vi "main.vi"() -> ()   [LabVIEW 2021]
uses:
  <vilib>/httpClient/LabVIEWHTTPClient.lvlib
  <vilib>/Analysis/NI_AALBase.lvlib
panel:
  out "数组":dbl[](array[numeric])
  in  "管理界面":bool
  in  "退出系统":bool
  in  "登录界面":bool
  in  "主界面":bool
  in  "选项卡":enum32{"主界面", "管理界面", "登录界面"}(tab)
  out "液位高度":dbl format="%#.1f"
  in  "请输入测量点高度":dbl
  out "测量点至水面距离":dbl format="%#.1f"
  in  "开关":bool
  out "液位过低":bool
  out "液位曲线图":dbl(graph)
  out "液位过高":bool
  out "实时液位":dbl(slide) scale=0.0..1000.0
  in  "密码组":string[](array[string])=["001", "002", "003"]
  in  "取消按钮":bool
  in  "登录按钮":bool=TRUE
  in  "密码":string
  in  "用户":enum16{"操作员", "管理员", "开发者"}(ring)
  # "超声波液位测量系统\n超声波液位测量系统"
  # "mm"
  # "mm"
  # "mm"
  # "mm"
  # "操作员"
  # "管理员"
  # "开发者"
  # "用户"
  # "密码"
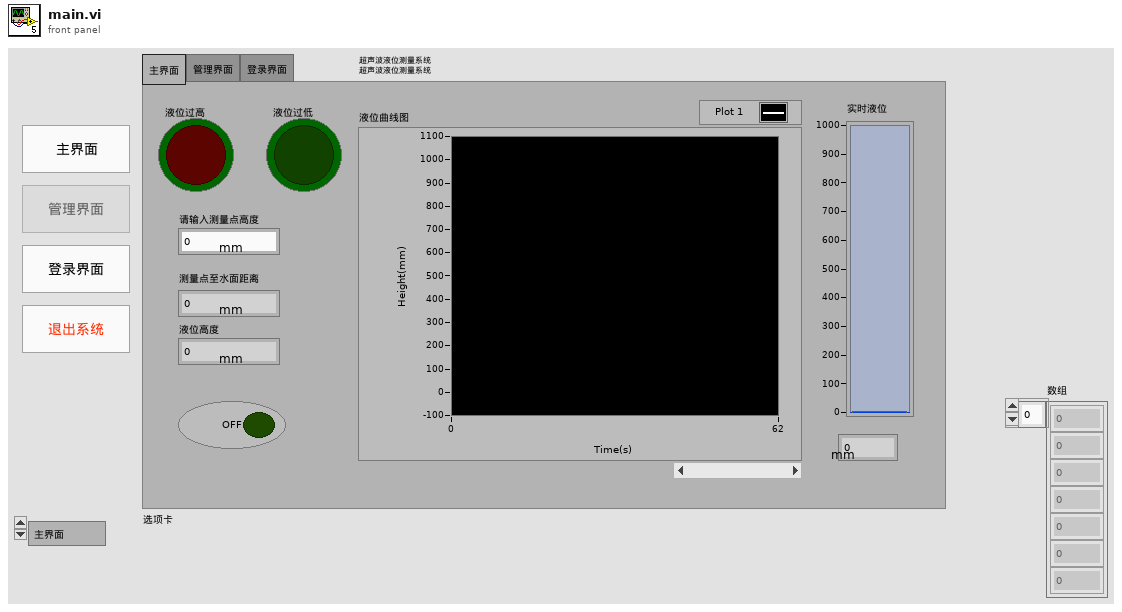
[diagram p1: front panel]
types:
  T1 = enum8{"Enabled", "Disabled", "Disabled and Grayed Out"}
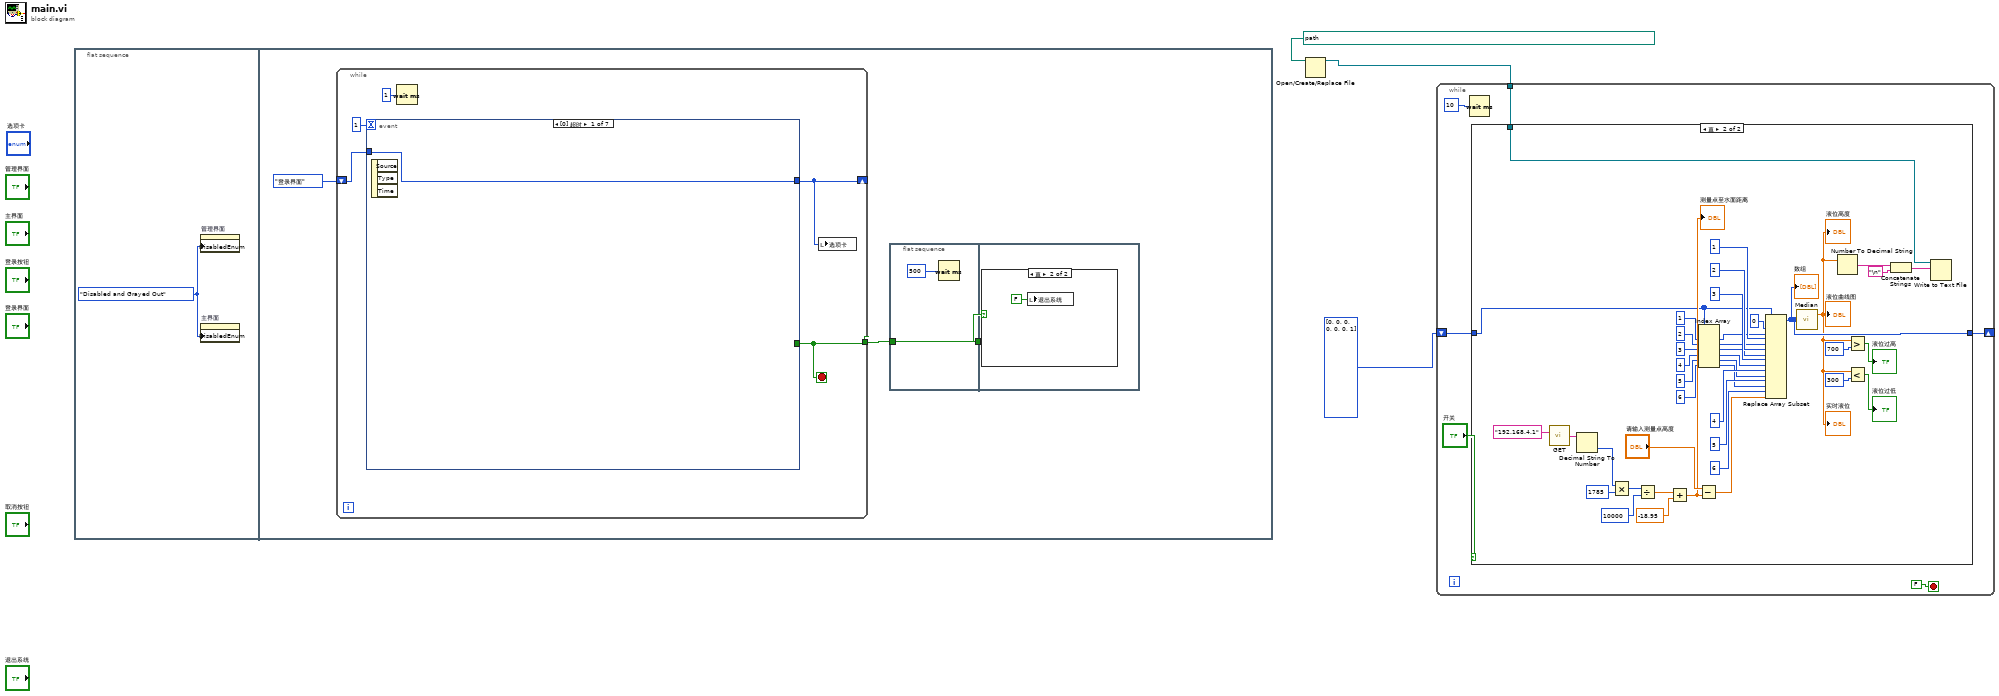
[diagram p0: block diagram]
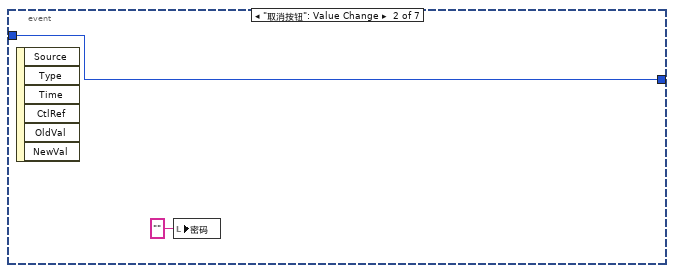
[diagram p4: hidden frame]
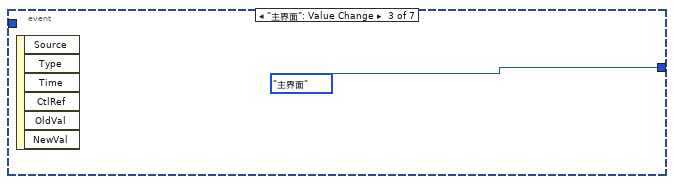
[diagram p5: hidden frame]
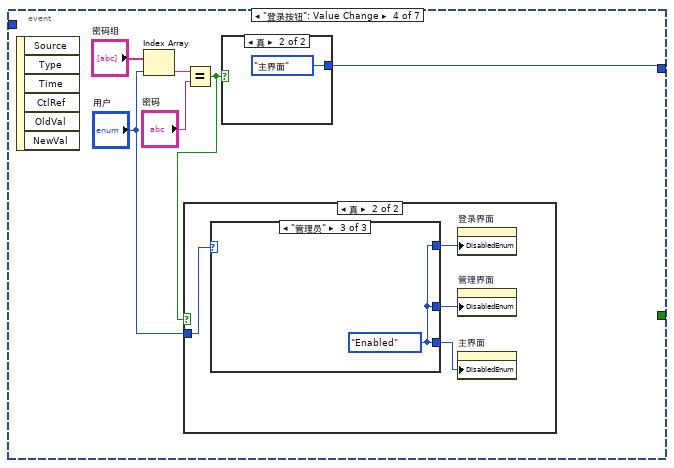
[diagram p6: hidden frame]
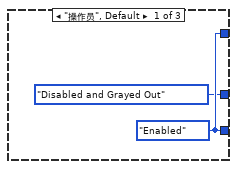
[diagram p8: hidden frame]
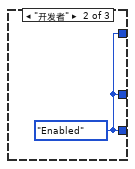
[diagram p9: hidden frame]
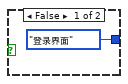
[diagram p10: hidden frame]
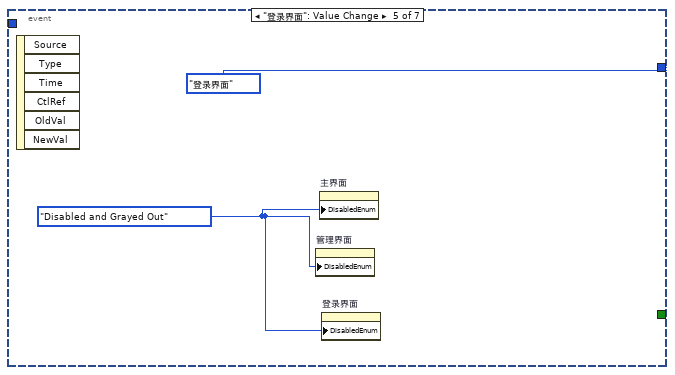
[diagram p11: hidden frame]
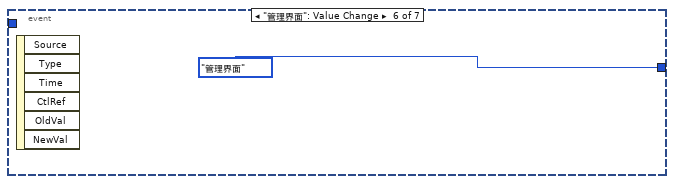
[diagram p12: hidden frame]
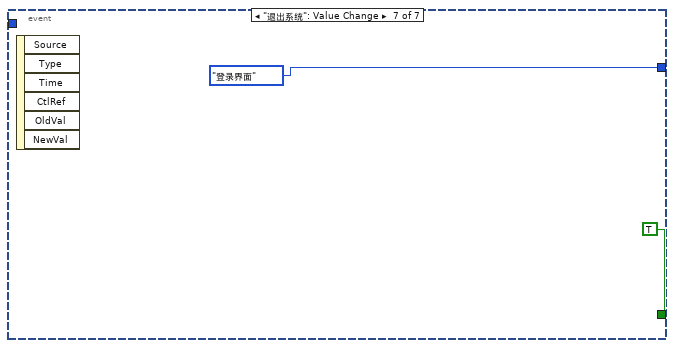
[diagram p13: hidden frame]
diagram:
  n1 = flat-sequence {
    frame #0 {
      w4 = T1."Disabled and Grayed Out" ("禁用")
      n2 = property on="管理界面" class="Bool (严格)"("DisabledEnum"=w4) -> ()  [unwired: 2 in, 2 out]
      n3 = property on="主界面" class="Bool (严格)"("DisabledEnum"=w4) -> ()  [unwired: 2 in, 2 out]
    }
    frame #1 {
      n4 = while {
        shift-right: [w12] -> _
        shift-left: enum32{"主界面", "管理界面", "登录界面"}."登录界面" ("选项卡") -> [w14]
        tunnel: [w13] -> w6
        stop <- w13 stop-if-true
        n5 = event shown="[0] 超时" {
          selector: _ -> [_ _ _ _ _ _ _]
          dyn-events: _ -> [_ _ _ _ _ _ _]
          timeout: 1 -> [_ _ _ _ _ _ _]
          tunnel: w14 -> [w17 w18 _ _ _ _ _]
          tunnel: [w17 w18 enum32{"主界面", "管理界面", "登录界面"}."主界面" ("选项卡") w23 enum32{"主界面", "管理界面", "登录界面"}."登录界面" ("选项卡") enum32{"主界面", "管理界面", "登录界面"}."管理界面" ("选项卡") enum32{"主界面", "管理界面", "登录界面"}."登录界面" ("选项卡")] -> w12
          tunnel: [_ _ _ _ _ _ TRUE] -> w13
          event Timeout {
            n6 = event-data() -> ()  [unwired: 1 in, 3 out]
          }
          event "取消按钮": Value Change {
            n7 = event-data() -> ()  [unwired: 1 in, 6 out]
            n8 = local write "密码"("" ("密码")) -> ()
          }
          event "主界面": Value Change {
            n9 = event-data() -> ()  [unwired: 1 in, 6 out]
          }
          event "登录按钮": Value Change {
            n10 = event-data() -> ()  [unwired: 1 in, 6 out]
            n11 = Index Array(array="密码组", index="用户") -> (element=w25:string)
            n12 = Equal?(x=w25, y="密码") -> (x = y?=w21:bool)
            n13 = case shown="真" w21 {
              tunnel: "用户" -> [_ w30]
              frame False {
              }
              frame True {
                n14 = case shown="\"管理员\"" w30 {
                  tunnel: [w32 w33 w34] -> w29
                  tunnel: [w32 w33 w34] -> w28
                  tunnel: [T1."Disabled and Grayed Out" ("禁用") w33 w34] -> w27
                  frame "操作员", Default {
                    w32 = T1."Enabled" ("禁用")
                  }
                  frame "开发者" {
                    w33 = T1."Enabled" ("禁用")
                  }
                  frame "管理员" {
                    w34 = T1."Enabled" ("禁用")
                  }
                }
                n15 = property on="登录界面" class="Bool (严格)"("DisabledEnum"=w28) -> ()  [unwired: 2 in, 2 out]
                n16 = property on="管理界面" class="Bool (严格)"("DisabledEnum"=w27) -> ()  [unwired: 2 in, 2 out]
                n17 = property on="主界面" class="Bool (严格)"("DisabledEnum"=w29) -> ()  [unwired: 2 in, 2 out]
              }
            }
            n18 = case shown="真" w21 {
              tunnel: [enum32{"主界面", "管理界面", "登录界面"}."登录界面" ("选项卡") enum32{"主界面", "管理界面", "登录界面"}."主界面" ("选项卡")] -> w23
              frame False {
              }
              frame True {
              }
            }
          }
          event "登录界面": Value Change {
            w37 = T1."Disabled and Grayed Out" ("禁用")
            n19 = event-data() -> ()  [unwired: 1 in, 6 out]
            n20 = property on="管理界面" class="Bool (严格)"("DisabledEnum"=w37) -> ()  [unwired: 2 in, 2 out]
            n21 = property on="主界面" class="Bool (严格)"("DisabledEnum"=w37) -> ()  [unwired: 2 in, 2 out]
            n22 = property on="登录界面" class="Bool (严格)"("DisabledEnum"=w37) -> ()  [unwired: 2 in, 2 out]
          }
          event "管理界面": Value Change {
            n23 = event-data() -> ()  [unwired: 1 in, 6 out]
          }
          event "退出系统": Value Change {
            n24 = event-data() -> ()  [unwired: 1 in, 6 out]
          }
        }
        n25 = Wait (ms)(milliseconds to wait=u32 1 ("等待时间（毫秒）")) -> ()  [unwired: 1 out]
        n26 = local write "选项卡"(w12) -> ()
      }
      n27 = flat-sequence {
        tunnel: w6 -> [w9]
        tunnel: [w9] -> w7
        tunnel: w7 -> [w10]
        frame #0 {
          n28 = Wait (ms)(milliseconds to wait=u32 500 ("毫秒计时值")) -> ()  [unwired: 1 out]
        }
        frame #1 {
          n29 = case shown="真" w10 {
            frame False {
            }
            frame True {
              n30 = local write "退出系统"(FALSE ("退出系统")) -> ()
            }
          }
        }
      }
    }
  }
  n31 = Open/Create/Replace File(file path (use dialog)=path "D:/Users/.comberdare/Desktop/超声波测量系统 文件夹/超声波测量系统 文件夹/Database.txt") -> (refnum out=w2:refnum<file>)  [unwired: 5 in, 2 out]
  n32 = while {
    tunnel: w2 -> [w44]
    shift-right: [w42] -> _
    shift-left: i32[] [0, 0, 0, 0, 0, 0, 1] -> [w43]
    stop <- FALSE stop-if-true
    n33 = Wait (ms)(milliseconds to wait=u32 10) -> ()  [unwired: 1 out]
    n34 = case shown="真" "开关" {
      tunnel: w44 -> [_ w89]
      tunnel: w43 -> [w48 w61]
      tunnel: [w48 w53] -> w42
      frame False {
      }
      frame True {
        n35 = call <vilib>:"GET.vi"("url"="192.168.4.1") -> ("body"=w51:string)  [unwired: 11 in, 3 out]
        n36 = Decimal String To Number(string=w51) -> (number=w49:i32)  [unwired: 2 in, 1 out]
        n37 = Multiply(x=w49, y=1785) -> (x*y=w86:i32)
        n38 = Divide(x=w86, y=10000) -> (x/y=w84:dbl)
        n39 = Add(x=w84, y=-18.95) -> (x+y=w82:dbl)
        "测量点至水面距离" <- w82
        n40 = Subtract(x="请输入测量点高度", y=w82) -> (x-y=w62:dbl)
        n41 = Index Array(array=w61, index #1=1 ("索引"), index #2=2 ("索引"), index #3=3 ("索引"), index #4=4 ("索引"), index #5=5 ("索引"), index #6=6 ("索引")) -> (element #1=w68:i32, element #2=w67:i32, element #3=w66:i32, element #4=w65:i32, element #5=w64:i32, element #6=w63:i32)
        n42 = Replace Array Subset(array=w61, new element #1=w68, index #1=0 ("索引"), new element #2=w67, index #2=1 ("索引"), new element #3=w66, index #3=2 ("索引"), new element #4=w65, index #4=3 ("索引"), new element #5=w64, index #5=4 ("索引"), new element #6=w63, index #6=5 ("索引"), new element #7=w62, index #7=6 ("索引")) -> (w53:i32[])
        "数组" <- w53
        n43 = call <vilib>:"Median.vi"("X"=w53) -> ("median"=w52:dbl)  [unwired: 1 out]
        "液位曲线图" <- w52
        "实时液位" <- w52
        "液位高度" <- w52
        n44 = Number To Decimal String(number=w52) -> (decimal integer string=w54:string)  [unwired: 1 in]
        n45 = Greater?(x=w52, y=700) -> (0:→"液位过高":bool)
        n46 = Less?(x=w52, y=300) -> (x < y?=→"液位过低":bool)
        n47 = Concatenate Strings(w54, "\n") -> (w55:string)
        n48 = Write to Text File(file (use dialog)=w89, text=w55) -> ()  [unwired: 2 in, 3 out]
      }
    }
  }
